vi "GPIB INIT & Clear.vi"(1 "error in":errorcluster, 2 "GPIB Address":i16) -> (0 "error out":errorcluster)   [LabVIEW 2019]
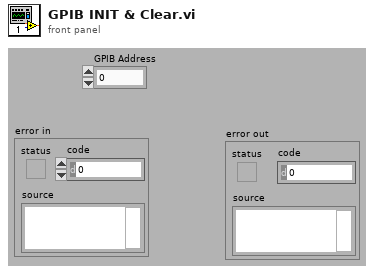
[diagram p1: front panel]
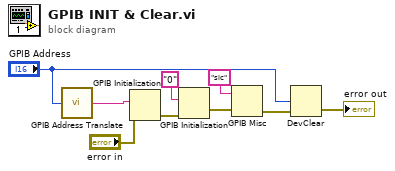
[diagram p0: block diagram]
diagram:
  n1 = call "GPIB Address Translate.vi"("GPIB Address"="GPIB Address") -> ("GPIB Address String"=w8:string)
  n2 = GPIB Initialization(4:"error in", 6:w8) -> (0:w3:errorcluster)  [unwired: 5 in]
  n3 = GPIB Initialization(4:w3, 6:"0" ("address string")) -> (0:w2:errorcluster)  [unwired: 5 in]
  n4 = GPIB Misc(0:"sic", 1:w2) -> (4:w7:errorcluster)  [unwired: 2 out]
  n5 = DevClear(2:w7, 3:"GPIB Address") -> (0:→"error out":errorcluster)  [unwired: 1 in, 1 out]
